vi "GenerateWavFilePath.vi"(8 "error in (no error)":errorcluster, 9 "center frequency":dbl, 10 "Channel Name":string, 11 "config":T1) -> (0 "error out":errorcluster, 3 "wav file path":path)   [LabVIEW 2017, in "EmsaAudio.lvlib"]
uses:
  <vilib>/addons/InsightCM/Devices/Shared/Emsa/EmsaAudio/EmsaAudio.lvlib
  <vilib>/addons/InsightCM/Devices/Shared/Emsa/EmsaAudio/controls/config.ctl
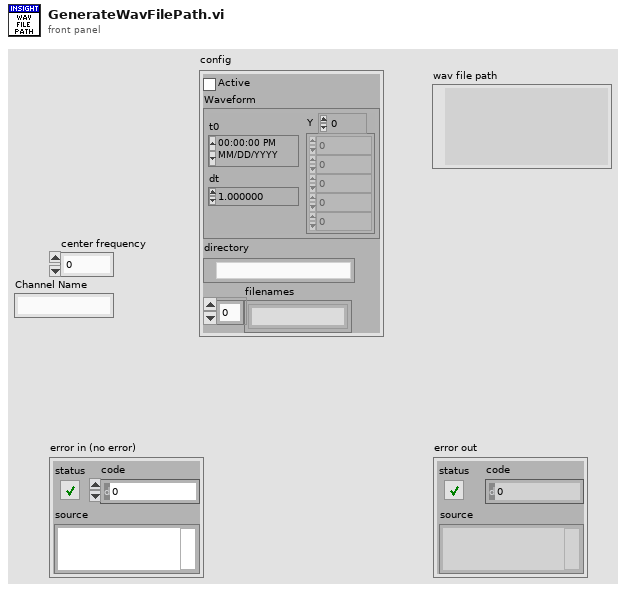
[diagram p1: front panel]
types:
  T1 = typedef "EmsaAudio.lvlib/config.ctl" = cluster{"Active":bool, "Waveform":waveform(dbl), "directory":path, "filenames":string[]}
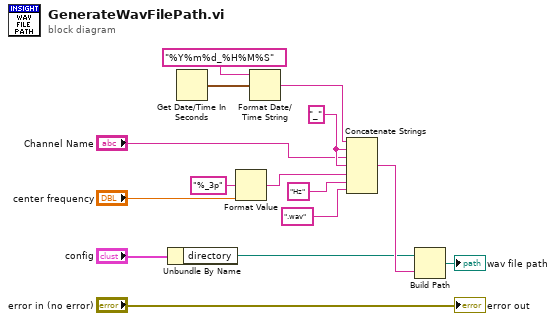
[diagram p0: block diagram]
diagram:
  w8 = "_" ("string")
  n1 = Unbundle By Name("config") -> ("directory"=w3:path)
  n2 = Get Date/Time In Seconds() -> (seconds since 1Jan1904=w11:timestamp)
  n3 = Format Value(format string="%_3p", value (0)="center frequency") -> (output string=w14:string)  [unwired: 1 in]
  n4 = Format Date/Time String(time format string (%c)="%Y%m%d_%H%M%S", seconds (now)=w11) -> (date/time string=w7:string)  [unwired: 1 in]
  n5 = Concatenate Strings(w7, w8, "Channel Name", w8, w14, "Hz" ("string"), ".wav" ("string")) -> (w10:string)
  n6 = Build Path(base path=w3, name or relative path=w10) -> (appended path=→"wav file path":path)
  "error out" <- "error in (no error)"
